vi "Gripper Control Loop.vi"() -> ()   [LabVIEW 2014, in "Elevator System.lvlib"]
uses:
  Elevator System.lvlib
  <vilib>/Rock Robotics/WPI/MotorControl/WPI_MotorControlDeviceRef.ctl
  <vilib>/Rock Robotics/WPI/MotorControl/WPI_MotorControlType.ctl
  <vilib>/Rock Robotics/SystemInterfaces/Typedef/FPGA_TypedefDigitalModule.ctl
  <vilib>/Rock Robotics/SystemInterfaces/DIO/FPGA_DIOPWMChannel.ctl
  <vilib>/Rock Robotics/WPI/PWM/WPI_PWMDeadband.ctl
  <vilib>/Rock Robotics/WPI/CAN/Jaguar/SubVIs/WPI_CANJaguar_ControlMode.ctl
  <vilib>/Rock Robotics/WPI/CAN/TalonSRX/WPI_CANTalonSRX_APIControlMode.ctl
  <vilib>/Rock Robotics/WPI/PWM/WPI_PWMTransform_ConPane.ctl
  Typedef/GripperNotifierType.ctl
  Public/Sensors Global.vi
  <vilib>/addons/control/pid/pid.llb/PID (DBL).vi
  <vilib>/addons/control/pid/NI_PID_pid.lvlib
panel:
  out "Plant Input":dbl(graph)
  in  "output range":cluster{"output high":dbl, "output low":dbl}={"output high"=1.0, "output low"=-1.0} {"output low" format="%.2f"; "output high" format="%.2f"}
  in  "PID gains":T1={"proportional gain (Kc)"=11.9, "integral time (Ti, min)"=0.004, "derivative time (Td, min)"=0.0} {"derivative time (Td, min)" format="%.3f"; "integral time (Ti, min)" format="%.3f"; "proportional gain (Kc)" format="%.3f"}
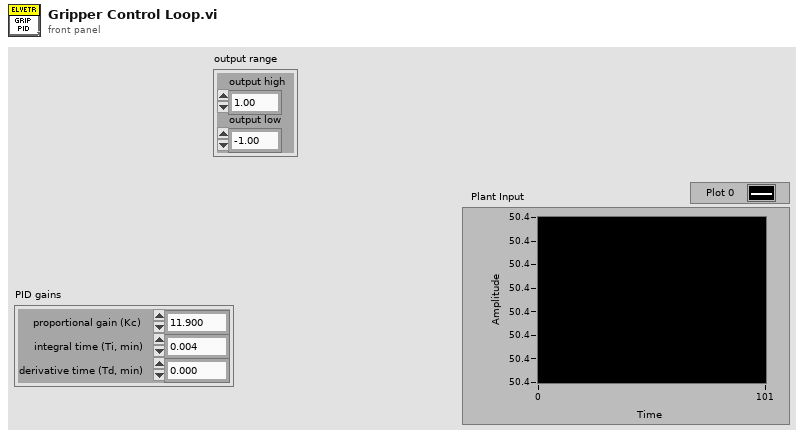
[diagram p1: front panel]
types:
  T1 = cluster{"proportional gain (Kc)":dbl, "integral time (Ti, min)":dbl, "derivative time (Td, min)":dbl}
  T2 = typedef "WPI_MotorControlDeviceRef.ctl" = cluster{"DeviceStatus":errorcluster, "Type":T3, "PWM":cluster{"Controller":T4, "PWM Channel":T5, "DeadBand":T6}, "CAN":cluster{"Device Number":u8, "Control Mode":T7, "Semaphore":T8, "Max Vout":dbl, "TalonSRX Control Mode":T9}, "Invert":bool, "TransformRef":T10, "InvTransformRef":T10}
  T3 = typedef "WPI_MotorControlType.ctl" = enum16{"PWM", "CAN", "CANTalonSRX"}
  T4 = typedef "FPGA_TypedefDigitalModule.ctl" = enum16{"Controller 1"}
  T5 = typedef "FPGA_DIOPWMChannel.ctl" = enum8{"PWM 0", "PWM 1", "PWM 2", "PWM 3", "PWM 4", "PWM 5", "PWM 6", "PWM 7", "PWM 8", "PWM 9", "PWM MXP 0", "PWM MXP 1", "PWM MXP 2", "PWM MXP 3", "PWM MXP 4", "PWM MXP 5", "PWM MXP 6", "PWM MXP 7", "PWM MXP 8", "PWM MXP 9", "Invalid"}
  T6 = typedef "WPI_PWMDeadband.ctl" = cluster{"Name":string, "maxPositivePwm":i32, "minPositivePwm":i32, "centerPwm":i32, "maxNegativePwm":i32, "minNegativePwm":i32, "angularRange":u16}
  T7 = typedef "WPI_CANJaguar_ControlMode.ctl" = enum8{"Percent VBus", "Current", "Speed", "Position", "Voltage"}
  T8 = typedef "Semaphore RefNum" = refnum<k1>
  T9 = typedef "WPI_CANTalonSRX_APIControlMode.ctl" = enum8{"Percent VBus", "Speed", "Position", "Slave", "Unchanged / Invalid"}
  T10 = typedef "WPI_PWMTransform_ConPane.ctl" = refnum<vi>
  T11 = typedef "Elevator System.lvlib/GripperNotifierType.ctl" = cluster{"SP Left":dbl, "SP Right":dbl}
  T12 = cluster{"Output":dbl, "GripperMotorL":T2, "GripperMotorR":T2, "notifier":refnum<notifier>, "Setpoint":T11}
  T13 = cluster{"static gain":dbl, "lag (s)":dbl, "deadtime (s)":dbl, "load":dbl, "deadband":dbl, "sensor noise":dbl, "initial PV":dbl, "plant noise":dbl}
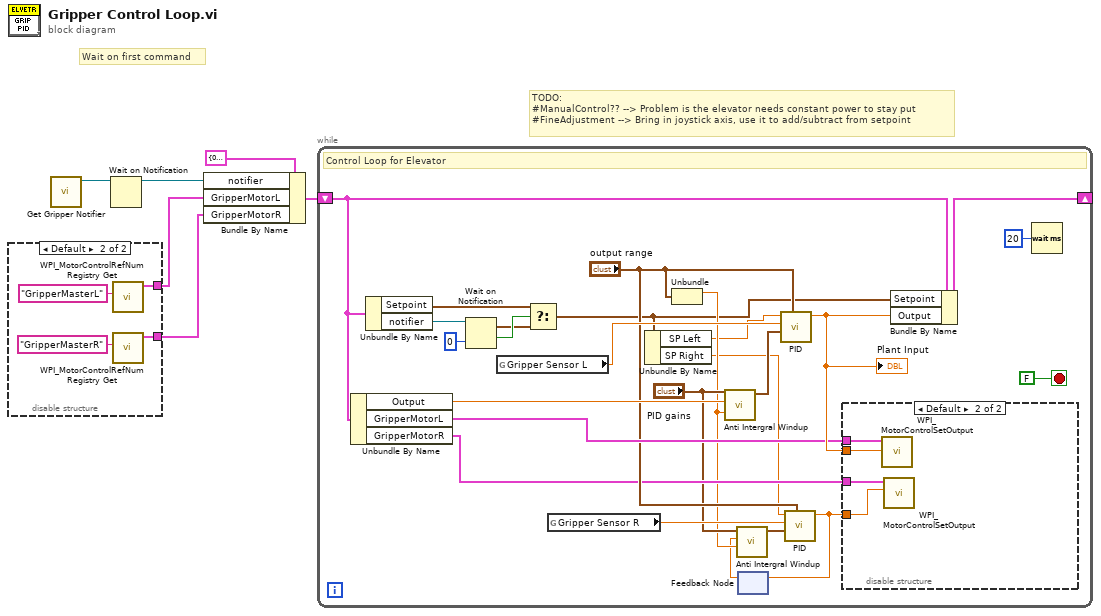
[diagram p0: block diagram]
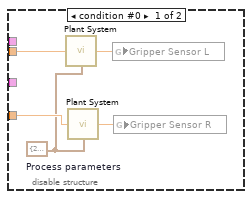
[diagram p3: hidden frame]
diagram:
  # "Wait on first command"
  # "TODO:\n#ManualControl?? --> Problem is the elevator needs constant power to stay put\n#FineAdjustment --> Bring in joystick axis, use it to add/subtract from setpoint"
  n1 = disable-structure shown="Default" {
    disable-tunnel: [_ w10] -> w5
    disable-tunnel: [_ w7] -> w4
    frame condition #0 {
    }
    frame condition #1 (active) {
      n2 = call <vilib>:"WPI_MotorControlRefNum Registry Get.vi"("refnum name"="GripperMasterL") -> ("MotorControlDevRef"=w10:T2)  [unwired: 9 in, 1 out]
      n3 = call <vilib>:"WPI_MotorControlRefNum Registry Get.vi"("refnum name"="GripperMasterR") -> ("MotorControlDevRef"=w7:T2)  [unwired: 9 in, 1 out]
    }
  }
  n4 = call "Get Gripper Notifier.vi"() -> ("Notifier out"=w3:refnum<notifier>)  [unwired: 11 in]
  n5 = Wait on Notification(notifier=w3) -> (notifier out=w1:refnum<notifier>)  [unwired: 3 in, 3 out]
  n6 = Bundle By Name(cluster=T12 {"Output"=0.0, "GripperMotorL"={"DeviceStatus"={"status"=FALSE, "code"=0, "source"=""}, "Type"=enum."PWM", "PWM"={"Controller"=enum."Controller 1", "PWM Channel"=enum."Invalid", "DeadBand"={"Name"="", "maxPositivePwm"=0, "minPositivePwm"=0, "centerPwm"=0, "maxNegativePwm"=0, "minNegativePwm"=0, "angularRange"=0}}, "CAN"={"Device Number"=0, "Control Mode"=enum."Percent VBus", "Semaphore"=refnum, "Max Vout"=12.0, "TalonSRX Control Mode"=enum."Percent VBus"}, "Invert"=FALSE, "TransformRef"=refnum, "InvTransformRef"=refnum}, "GripperMotorR"={"DeviceStatus"={"status"=FALSE, "code"=0, "source"=""}, "Type"=enum."PWM", "PWM"={"Controller"=enum."Controller 1", "PWM Channel"=enum."Invalid", "DeadBand"={"Name"="", "maxPositivePwm"=0, "minPositivePwm"=0, "centerPwm"=0, "maxNegativePwm"=0, "minNegativePwm"=0, "angularRange"=0}}, "CAN"={"Device Number"=0, "Control Mode"=enum."Percent VBus", "Semaphore"=refnum, "Max Vout"=12.0, "TalonSRX Control Mode"=enum."Percent VBus"}, "Invert"=FALSE, "TransformRef"=refnum, "InvTransformRef"=refnum}, "notifier"=refnum, "Setpoint"={"SP Left"=0.0, "SP Right"=0.0}}, "notifier"=w1, "GripperMotorL"=w5, "GripperMotorR"=w4) -> (w6:T12)
  n7 = while {
    shift-right: [w30] -> _
    shift-left: w6 -> [w29]
    stop <- FALSE stop-if-true
    # "Control Loop for Elevator"
    n8 = Unbundle By Name(w29) -> ("Output"=w28:dbl, "GripperMotorL"=w22:T2, "GripperMotorR"=w19:T2)
    n9 = Unbundle By Name(w29) -> ("Setpoint"=w32:T11, "notifier"=w34:refnum<notifier>)
    n10 = Wait on Notification(notifier=w34, timeout in ms (-1)=0) -> (notification=w24:T11, timed out?=w33:bool)  [unwired: 2 in, 2 out]
    n11 = global read "Sensors Global.vi" "Gripper Sensor L"() -> (w27:dbl)
    n12 = Select(t=w32, s=w33, f=w24) -> (s? t:f=w13:T11)
    n13 = global read "Sensors Global.vi" "Gripper Sensor R"() -> (w20:dbl)
    n14 = Unbundle By Name(w13) -> ("SP Left"=w12:dbl, "SP Right"=w11:dbl)
    n15 = Unbundle("output range") -> ("output high"=w16:dbl)  [unwired: 1 out]
    n16 = call "Anti Intergral Windup.vi"("|Limit|"=w16, "MV"=w28, "PID gains"="PID gains") -> ("PID gains"=w31:T1)  [unwired: 8 in]
    n17 = feedback #1() -> (w14:dbl)  [unwired: 1 in]
    n18 = call "Anti Intergral Windup.vi"("|Limit|"=w16, "MV"=w14, "PID gains"="PID gains") -> ("PID gains"=w17:T1)  [unwired: 8 in]
    n19 = call-poly <vilib>:"PID.vi"("output range"="output range", "PID gains"=w31, "process variable"=w27, "setpoint"=w12) -> ("output"=w23:dbl)  [unwired: 6 in, 1 out]
    "Plant Input" <- w23
    n20 = call-poly <vilib>:"PID.vi"("output range"="output range", "PID gains"=w17, "process variable"=w20, "setpoint"=w11) -> ("output"=w15:dbl)  [unwired: 6 in, 1 out]
    n21 = feedback-in #1(w15) -> ()
    n22 = disable-structure shown="Default" {
      disable-tunnel: w23 -> [w40 w44]
      disable-tunnel: w22 -> [_ w43]
      disable-tunnel: w19 -> [_ w42]
      disable-tunnel: w15 -> [w37 w41]
      frame condition #0 {
        w36 = T13 {"static gain"=2.5, "lag (s)"=2.5, "deadtime (s)"=0.01, "load"=40.0, "deadband"=0.0, "sensor noise"=0.0, "initial PV"=0.0, "plant noise"=0.0}  # Process parameters
        n23 = call "Plant System.vi"("Plant Input"=w40, "process parameters"=w36) -> ("Plant Output"=w39:dbl)  [unwired: 13 in]
        n24 = call "Plant System.vi"("Plant Input"=w37, "process parameters"=w36) -> ("Plant Output"=w38:dbl)  [unwired: 13 in]
        n25 = global write "Sensors Global.vi" "Gripper Sensor L"(w39) -> ()
        n26 = global write "Sensors Global.vi" "Gripper Sensor R"(w38) -> ()
      }
      frame condition #1 (active) {
        n27 = call <vilib>:"WPI_MotorControlSetOutput.vi"("Output"=w44, "MotorControlDevRef"=w43) -> ()  [unwired: 7 in, 3 out]
        n28 = call <vilib>:"WPI_MotorControlSetOutput.vi"("Output"=w41, "MotorControlDevRef"=w42) -> ()  [unwired: 7 in, 3 out]
      }
    }
    n29 = Bundle By Name(cluster=w29, "Setpoint"=w13, "Output"=w23) -> (w30:T12)
    n30 = Wait (ms)(milliseconds to wait=u32 20) -> ()  [unwired: 1 out]
  }
